vi "H5Pset_fapl_split.vi"(4 "Raw Extension":string, 5 "Meta Extension":string, 6 "error in (no error)":errorcluster, 7 "Raw Property List":T1, 8 "Meta Property List":T1, 9 "HDF5 Property List Ref":T1) -> (0 "error out":errorcluster, 3 "HDF5 Property List Ref out":T1)   [LabVIEW 2017]
doc: "Emulates the old split file driver."
uses:
  <vilib>/UPVI/lvhdf5/library.llb/HDF5 Ref.ctl
  <vilib>/UPVI/lvhdf5/hdf5.dll
panel:
  # "LVHDF5 Toolkit\nCopyright (c) 2005-2013 by Jason D. Sommerville\nCopyright (c) 2014 by UPVI, LLC.\n\nThis use and distribution of this file is governed by the terms found in \nLICENSE.txt distributed with this toolkit and installed at\n <user.lib>\\_lvhdf5\\LICENSE.txt"
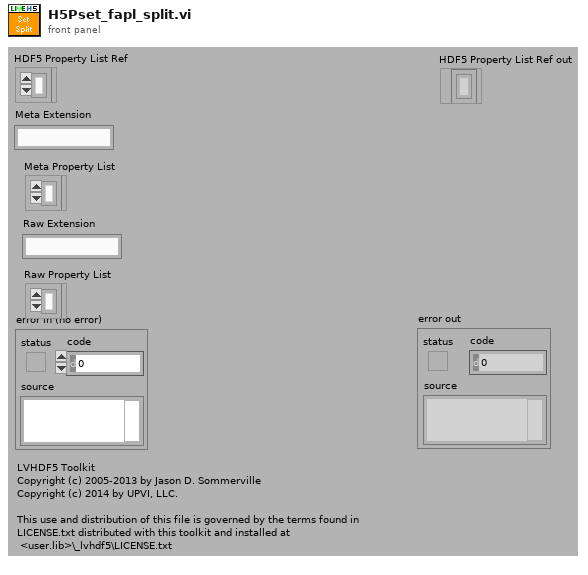
[diagram p1: front panel]
types:
  T1 = typedef "HDF5 Ref.ctl" = refnum<k1>
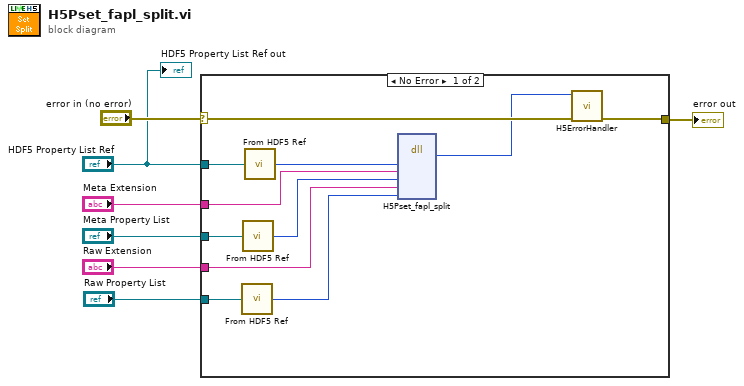
[diagram p0: block diagram]
diagram:
  n1 = case shown="No Error" "error in (no error)" {
    selector: "error in (no error)" -> [w18 w19]
    tunnel: [w17 w19] -> w6
    tunnel: "HDF5 Property List Ref" -> [w16 _]
    tunnel: "Meta Extension" -> [w13 _]
    tunnel: "Meta Property List" -> [w12 _]
    tunnel: "Raw Property List" -> [w11 _]
    tunnel: "Raw Extension" -> [w9 _]
    frame No Error {
      n2 = call <vilib>:"From HDF5 Ref.vi"("HDF5 Ref"=w11) -> ("I32"=w8:i32)
      n3 = call <vilib>:"From HDF5 Ref.vi"("HDF5 Ref"=w12) -> ("I32"=w10:i32)
      n4 = call <vilib>:"From HDF5 Ref.vi"("HDF5 Ref"=w16) -> ("I32"=w15:i32)
      n5 = dll-call lib="C:/Program Files/National Instruments/LabVIEW 2017/vi.lib/UPVI/lvhdf5/hdf5.dll" fn="H5Pset_fapl_split"("plist_id"=w15, "meta_ext"=w13, "meta_plist_id"=w10, "raw_ext"=w9, "raw_plist_id"=w8) -> (w14:i32)  [unwired: 8 in, 2 out]
      n6 = call <vilib>:"H5ErrorHandler.vi"("error in (no error)"=w18, "herr_t"=w14) -> ("error out"=w17:errorcluster)  [unwired: 3 in, 4 out]
    }
    frame Error {
    }
  }
  "error out" <- w6
  "HDF5 Property List Ref out" <- "HDF5 Property List Ref"
